vi "Teleop.vi"(10 "Match Info":T1={"Autonomous Elapsed Seconds"=0.0, "TeleOp Elapsed Seconds"=0.0, "Disabled Elapsed Seconds"=0.0, "Visited Autonomous"=FALSE, "Visited TeleOp"=FALSE, "Visited Disabled"=FALSE, "Autonomous Settings"={"Autonomous Style"=enum."Independent", "VI Refnum"=refnum}}, 11 "Call Context":T2) -> ()   [LabVIEW 2019]
doc: "This VI is called for each TeleOp packet received from the DS where the robot is not disabled. It is often used to read from the joysticks and update I/O or to update setpoints for timed control loops. It should complete and return within 20 milliseconds or it may miss DS packets."
uses:
  <vilib>/Rock Robotics/WPI/DriverStation/WPI_DriverStationDerivedRobotMode.ctl
  <vilib>/Rock Robotics/WPI/DriverStation/WPI_DriverStationMatch Info.ctl
  <vilib>/Rock Robotics/WPI/Utilities/WPI_GetSetVariantRefNum.vi
  <vilib>/Rock Robotics/Network Tables/NT Write Boolean Array.vi
  <vilib>/Rock Robotics/Network Tables/NT Write Numeric Array.vi
  <vilib>/Rock Robotics/Network Tables/NT Read Boolean.vi
  <vilib>/Rock Robotics/Network Tables/NT Read Number.vi
  <vilib>/Rock Robotics/Network Tables/NT Write Boolean.vi
  <vilib>/Rock Robotics/Network Tables/NT Write Number.vi
  <vilib>/Rock Robotics/Network Tables/NT Write String.vi
panel:
  out "Sample Slider 0":dbl(slide) scale=0.0..5.0
  out "Sample Boolean 1":bool
  out "Sample Boolean 0":bool
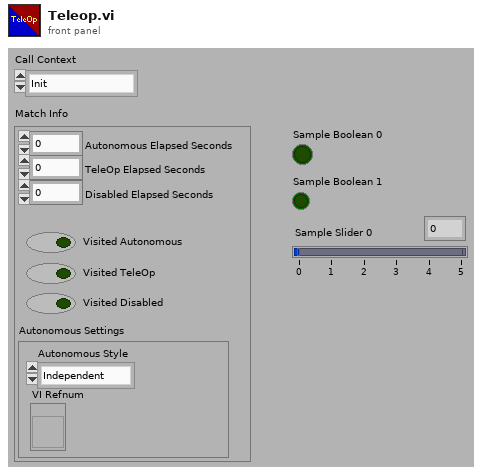
[diagram p1: front panel]
types:
  T1 = typedef "WPI_DriverStationMatch Info.ctl" = cluster{"Autonomous Elapsed Seconds":dbl, "TeleOp Elapsed Seconds":dbl, "Disabled Elapsed Seconds":dbl, "Visited Autonomous":bool, "Visited TeleOp":bool, "Visited Disabled":bool, "Autonomous Settings":cluster{"Autonomous Style":enum16{"Iterative", "Independent"}, "VI Refnum":refnum<vi>}}
  T2 = typedef "WPI_DriverStationDerivedRobotMode.ctl" = enum16{"Init", "Execute", "Stop"}
  T3 = typedef "WPI_JoystickDevRef.ctl" = cluster{"Device":T4}
  T4 = typedef "WPI_JoystickDeviceEnum.ctl" = enum16{"USB 0", "USB 1", "USB 2", "USB 3", "USB 4", "USB 5"}
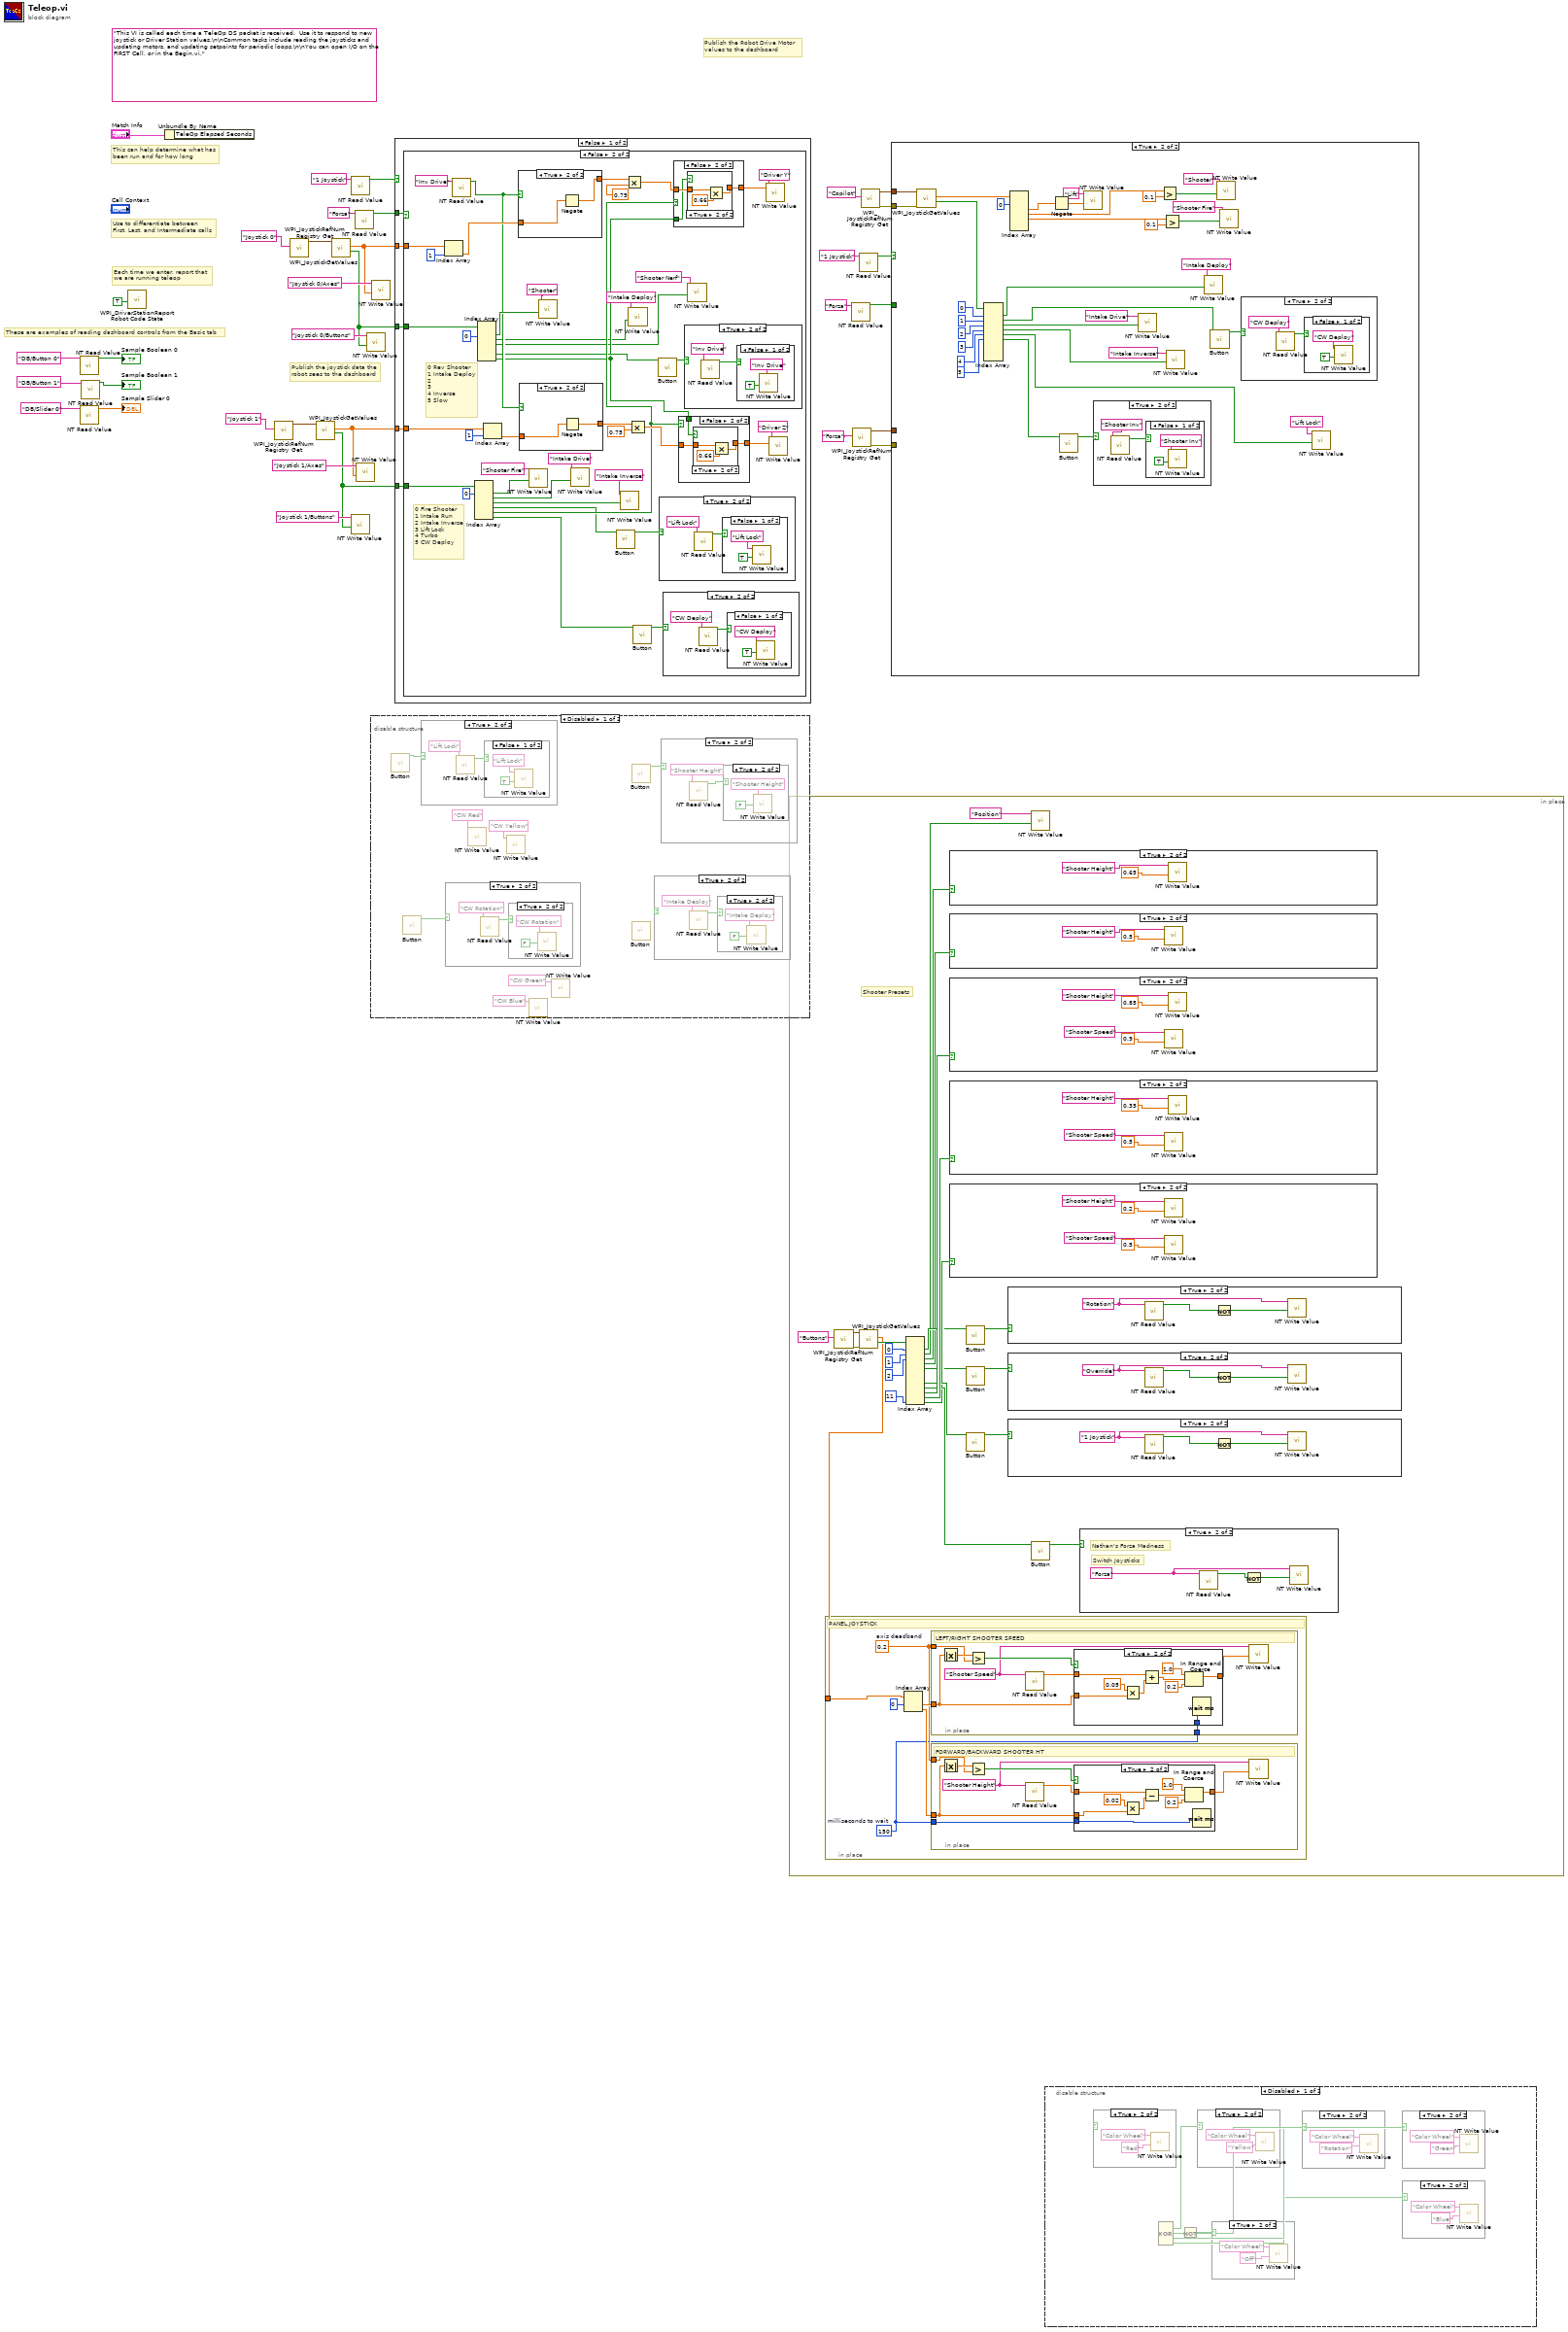
[diagram p0: block diagram]
diagram:
  (unwired) "This VI is called each time a TeleOp DS packet is received.  Use it to respond to new joystick or Driver Station values.\n\nCommon tasks include reading the joysticks and updating motors, and updating setpoints for periodic loops.\n\nYou can open I/O on the FIRST Call, or in the Begin.vi."
  # "These are examples of reading dashboard controls from the Basic tab"
  # "Publish the Robot Drive Motor\nvalues to the dashboard"
  # "Publish the joystick data the\nrobot sees to the dashboard"
  # "Each time we enter, report that\nwe are running teleop"
  # "Use to differentiate between\nFirst, Last, and Intermediate calls"
  # "This can help determine what has\nbeen run and for how long"
  n1 = call-poly <vilib>:"NT Read Value.vi"("Name"="DB/Button 0" ("refnum name")) -> ("Boolean"=→"Sample Boolean 0":bool)  [unwired: 9 in, 1 out]
  n2 = call-poly <vilib>:"NT Read Value.vi"("Name"="DB/Slider 0" ("refnum name")) -> ("Numeric"=→"Sample Slider 0":dbl)  [unwired: 9 in, 1 out]
  n3 = call-poly <vilib>:"NT Read Value.vi"("Name"="DB/Button 1" ("refnum name")) -> ("Boolean"=→"Sample Boolean 1":bool)  [unwired: 9 in, 1 out]
  n4 = call <vilib>:"WPI_DriverStationReport Robot Code State.vi"("TeleOp"=TRUE ("Autonomous")) -> ()  [unwired: 10 in, 1 out]
  n5 = Unbundle By Name("Match Info") -> ()  [unwired: 1 out]
  n6 = call <vilib>:"WPI_JoystickRefNum Registry Get.vi"("refnum name"="Joystick 1") -> ("JoystickDevRef"=w14:T3)  [unwired: 1 in, 9 out]
  n7 = call <vilib>:"WPI_JoystickRefNum Registry Get.vi"("refnum name"="Joystick 0") -> ("JoystickDevRef"=w32:T3)  [unwired: 1 in, 9 out]
  n8 = call <vilib>:"WPI_JoystickGetValues.vi"("JoystickDevRef"=w14) -> ("Buttons"=w10:bool[], "Axes"=w11:dbl[])  [unwired: 6 in, 3 out]
  n9 = call <vilib>:"WPI_JoystickGetValues.vi"("JoystickDevRef"=w32) -> ("Buttons"=w21:bool[], "Axes"=w28:dbl[])  [unwired: 6 in, 3 out]
  n10 = call-poly <vilib>:"NT Write Value.vi"("Boolean Array"=w10, "Name"="Joystick 1/Buttons") -> ()  [unwired: 9 in, 1 out]
  n11 = call-poly <vilib>:"NT Read Value.vi"("Name"="1 Joystick") -> ("Boolean"=w16:bool)  [unwired: 9 in, 1 out]
  n12 = call-poly <vilib>:"NT Read Value.vi"("Name"="Forza") -> ("Boolean"=w4:bool)  [unwired: 9 in, 1 out]
  n13 = call-poly <vilib>:"NT Write Value.vi"("Numeric Array"=w11, "Name"="Joystick 1/Axes") -> ()  [unwired: 9 in, 1 out]
  n14 = call-poly <vilib>:"NT Write Value.vi"("Boolean Array"=w21, "Name"="Joystick 0/Buttons") -> ()  [unwired: 9 in, 1 out]
  n15 = disable-structure shown="Disabled" {
    frame Disabled {
      n16 = call "Button.vi"() -> ("Button Pressed?"=w40:bool)  [unwired: 11 in]
      n17 = call "Button.vi"() -> ("Button Pressed?"=w35:bool)  [unwired: 11 in]
      n18 = case shown="True" w40 {
        frame False {
        }
        frame True {
          n19 = call-poly <vilib>:"NT Read Value.vi"("Name"="Lift Lock") -> ("Boolean"=w49:bool)  [unwired: 9 in, 1 out]
          n20 = case shown="False" w49 {
            frame False {
              n21 = call-poly <vilib>:"NT Write Value.vi"("Boolean"=TRUE, "Name"="Lift Lock") -> ()  [unwired: 9 in, 1 out]
            }
            frame True {
              n22 = call-poly <vilib>:"NT Write Value.vi"("Boolean"=FALSE, "Name"="Lift Lock") -> ()  [unwired: 9 in, 1 out]
            }
          }
        }
      }
      n23 = case shown="True" w35 {
        frame False {
        }
        frame True {
          n24 = call-poly <vilib>:"NT Read Value.vi"("Name"="CW Rotation") -> ("Boolean"=w43:bool)  [unwired: 9 in, 1 out]
          n25 = case shown="True" w43 {
            frame False {
              n26 = call-poly <vilib>:"NT Write Value.vi"("Boolean"=TRUE, "Name"="CW Rotation") -> ()  [unwired: 9 in, 1 out]
            }
            frame True {
              n27 = call-poly <vilib>:"NT Write Value.vi"("Boolean"=FALSE, "Name"="CW Rotation") -> ()  [unwired: 9 in, 1 out]
            }
          }
        }
      }
      n28 = call-poly <vilib>:"NT Write Value.vi"("Name"="CW Red") -> ()  [unwired: 10 in, 1 out]
      n29 = call-poly <vilib>:"NT Write Value.vi"("Name"="CW Yellow") -> ()  [unwired: 10 in, 1 out]
      n30 = call-poly <vilib>:"NT Write Value.vi"("Name"="CW Blue") -> ()  [unwired: 10 in, 1 out]
      n31 = call-poly <vilib>:"NT Write Value.vi"("Name"="CW Green") -> ()  [unwired: 10 in, 1 out]
      n32 = call "Button.vi"() -> ("Button Pressed?"=w42:bool)  [unwired: 11 in]
      n33 = call "Button.vi"() -> ()  [unwired: 11 in, 1 out]
      n34 = case shown="True" w41 {
        frame False {
        }
        frame True {
          n35 = call-poly <vilib>:"NT Read Value.vi"("Name"="Intake Deploy") -> ("Boolean"=w55:bool)  [unwired: 9 in, 1 out]
          n36 = case shown="True" w55 {
            frame False {
              n37 = call-poly <vilib>:"NT Write Value.vi"("Boolean"=TRUE, "Name"="Intake Deploy") -> ()  [unwired: 9 in, 1 out]
            }
            frame True {
              n38 = call-poly <vilib>:"NT Write Value.vi"("Boolean"=FALSE, "Name"="Intake Deploy") -> ()  [unwired: 9 in, 1 out]
            }
          }
        }
      }
      n39 = case shown="True" w42 {
        frame False {
        }
        frame True {
          n40 = call-poly <vilib>:"NT Read Value.vi"("Name"="Shooter Height") -> ("Boolean"=w61:bool)  [unwired: 9 in, 1 out]
          n41 = case shown="True" w61 {
            frame False {
              n42 = call-poly <vilib>:"NT Write Value.vi"("Boolean"=TRUE, "Name"="Shooter Height") -> ()  [unwired: 9 in, 1 out]
            }
            frame True {
              n43 = call-poly <vilib>:"NT Write Value.vi"("Boolean"=FALSE, "Name"="Shooter Height") -> ()  [unwired: 9 in, 1 out]
            }
          }
        }
      }
    }
    frame Enabled {
    }
  }
  n44 = call-poly <vilib>:"NT Write Value.vi"("Numeric Array"=w28, "Name"="Joystick 0/Axes") -> ()  [unwired: 9 in, 1 out]
  n45 = case shown="False" w16 {
    tunnel: w28 -> [w71 w179]
    tunnel: w21 -> [w70 w178]
    tunnel: w11 -> [w69 _]
    tunnel: w10 -> [w68 _]
    tunnel: w4 -> [w67 _]
    frame False {
      n46 = case shown="False" w67 {
        tunnel: w71 -> [_ w105]
        tunnel: w70 -> [_ w104]
        tunnel: w69 -> [_ w103]
        tunnel: w68 -> [_ w101]
        frame True {
        }
        frame False {
          # "0 Fire Shooter\n1 Intake Run\n2 Intake Inverse\n3 Lift Lock\n4 Turbo\n5 CW Deploy"
          # "0 Rev Shooter\n1 Intake Deploy\n2\n3\n4 Inverse\n5 Slow"
          n47 = Index Array(array=w105, index=1) -> (element=w110:dbl)
          n48 = call-poly <vilib>:"NT Read Value.vi"("Name"="Inv Drive") -> ("Boolean"=w84:bool)  [unwired: 9 in, 1 out]
          n49 = Index Array(array=w101, index #1=0 ("index")) -> (element #1=w92:bool, element #2=w89:bool, element #3=w77:bool, element #4=w78:bool, element #5=w83:bool, element #6=w86:bool)  [unwired: 5 in]
          n50 = Index Array(array=w104, index #1=0) -> (element #1=w88:bool, element #2=w74:bool, element #3=w72:bool, element #5=w81:bool, element #6=w80:bool)  [unwired: 5 in, 1 out]
          n51 = Index Array(array=w103, index=1) -> (element=w100:dbl)
          n52 = case shown="True" w84 {
            tunnel: w110 -> [w145 w147]
            tunnel: [w145 w146] -> w109
            frame False {
            }
            frame True {
              n53 = Negate(x=w147) -> (-x=w146:dbl)
            }
          }
          n54 = case shown="True" w84 {
            tunnel: w100 -> [w142 w144]
            tunnel: [w142 w143] -> w95
            frame False {
            }
            frame True {
              n55 = Negate(x=w144) -> (-x=w143:dbl)
            }
          }
          n56 = call-poly <vilib>:"NT Write Value.vi"("Boolean"=w92, "Name"="Shooter Fire") -> ()  [unwired: 9 in, 1 out]
          n57 = call-poly <vilib>:"NT Write Value.vi"("Boolean"=w88, "Name"="Shooter") -> ()  [unwired: 9 in, 1 out]
          n58 = call-poly <vilib>:"NT Write Value.vi"("Boolean"=w89, "Name"="Intake Drive") -> ()  [unwired: 9 in, 1 out]
          n59 = call "Button.vi"("Button In"=w78) -> ("Button Pressed?"=w79:bool)  [unwired: 10 in]
          n60 = call-poly <vilib>:"NT Write Value.vi"("Boolean"=w77, "Name"="Intake Inverse") -> ()  [unwired: 9 in, 1 out]
          n61 = Multiply(x=w109, y=0.75) -> (x*y=w108:dbl)
          n62 = call-poly <vilib>:"NT Write Value.vi"("Boolean"=w74, "Name"="Intake Deploy") -> ()  [unwired: 9 in, 1 out]
          n63 = Multiply(x=w95, y=0.75) -> (x*y=w98:dbl)
          n64 = call "Button.vi"("Button In"=w86) -> ("Button Pressed?"=w87:bool)  [unwired: 10 in]
          n65 = call "Button.vi"("Button In"=w81) -> ("Button Pressed?"=w82:bool)  [unwired: 10 in]
          n66 = case shown="True" w79 {
            frame False {
            }
            frame True {
              n67 = call-poly <vilib>:"NT Read Value.vi"("Name"="Lift Lock") -> ("Boolean"=w114:bool)  [unwired: 9 in, 1 out]
              n68 = case shown="False" w114 {
                frame False {
                  n69 = call-poly <vilib>:"NT Write Value.vi"("Boolean"=TRUE, "Name"="Lift Lock") -> ()  [unwired: 9 in, 1 out]
                }
                frame True {
                  n70 = call-poly <vilib>:"NT Write Value.vi"("Boolean"=FALSE, "Name"="Lift Lock") -> ()  [unwired: 9 in, 1 out]
                }
              }
            }
          }
          n71 = case shown="True" w87 {
            frame False {
            }
            frame True {
              n72 = call-poly <vilib>:"NT Read Value.vi"("Name"="CW Deploy") -> ("Boolean"=w126:bool)  [unwired: 9 in, 1 out]
              n73 = case shown="False" w126 {
                frame False {
                  n74 = call-poly <vilib>:"NT Write Value.vi"("Boolean"=TRUE, "Name"="CW Deploy") -> ()  [unwired: 9 in, 1 out]
                }
                frame True {
                  n75 = call-poly <vilib>:"NT Write Value.vi"("Boolean"=FALSE, "Name"="CW Deploy") -> ()  [unwired: 9 in, 1 out]
                }
              }
            }
          }
          n76 = case shown="False" w83 {
            tunnel: w108 -> [w149 w153]
            tunnel: [w148 w152] -> w107
            tunnel: w80 -> [_ w151]
            frame True {
              n77 = Multiply(x=w149, y=1.33) -> (x*y=w148:dbl)
            }
            frame False {
              n78 = case shown="True" w151 {
                tunnel: w153 -> [w154 w156]
                tunnel: [w154 w155] -> w152
                frame False {
                }
                frame True {
                  n79 = Multiply(x=w156, y=0.66) -> (x*y=w155:dbl)
                }
              }
            }
          }
          n80 = case shown="False" w83 {
            tunnel: w98 -> [w133 w137]
            tunnel: [w132 w136] -> w97
            tunnel: w80 -> [_ w135]
            frame True {
              n81 = Multiply(x=w133, y=1.33) -> (x*y=w132:dbl)
            }
            frame False {
              n82 = case shown="True" w135 {
                tunnel: w137 -> [w138 w140]
                tunnel: [w138 w139] -> w136
                frame False {
                }
                frame True {
                  n83 = Multiply(x=w140, y=0.66) -> (x*y=w139:dbl)
                }
              }
            }
          }
          n84 = case shown="True" w82 {
            frame False {
            }
            frame True {
              n85 = call-poly <vilib>:"NT Read Value.vi"("Name"="Inv Drive") -> ("Boolean"=w120:bool)  [unwired: 9 in, 1 out]
              n86 = case shown="False" w120 {
                frame False {
                  n87 = call-poly <vilib>:"NT Write Value.vi"("Boolean"=TRUE, "Name"="Inv Drive") -> ()  [unwired: 9 in, 1 out]
                }
                frame True {
                  n88 = call-poly <vilib>:"NT Write Value.vi"("Boolean"=FALSE, "Name"="Inv Drive") -> ()  [unwired: 9 in, 1 out]
                }
              }
            }
          }
          n89 = call-poly <vilib>:"NT Write Value.vi"("Boolean"=w72, "Name"="Shooter Nerf") -> ()  [unwired: 9 in, 1 out]
          n90 = call-poly <vilib>:"NT Write Value.vi"("Numeric"=w107, "Name"="Driver Y") -> ()  [unwired: 9 in, 1 out]
          n91 = call-poly <vilib>:"NT Write Value.vi"("Numeric"=w97, "Name"="Driver Z") -> ()  [unwired: 9 in, 1 out]
        }
      }
    }
    frame True {
      # "0 Turbo\n1 Slow\n2\n3\n4 Inverse\n5"
      n92 = Index Array(array=w179, index #1=1, index #2=3) -> (element #1=w173:dbl, element #2=w168:dbl)
      n93 = Index Array(array=w178, index #1=0) -> (element #1=w162:bool, element #2=w163:bool, element #5=w160:bool)  [unwired: 5 in, 3 out]
      n94 = call-poly <vilib>:"NT Read Value.vi"("Name"="Inv Drive") -> ("Boolean"=w159:bool)  [unwired: 9 in, 1 out]
      n95 = Multiply(x=w168, y=0.5) -> (x*y=w169:dbl)
      n96 = case shown="True" w159 {
        tunnel: w173 -> [w196 w198]
        tunnel: [w196 w197] -> w172
        frame False {
        }
        frame True {
          n97 = Negate(x=w198) -> (-x=w197:dbl)
        }
      }
      n98 = case shown="True" w162 {
        tunnel: [w186 w190] -> w167
        tunnel: w169 -> [w187 w191]
        tunnel: w163 -> [_ w189]
        frame True {
          n99 = Multiply(x=w187, y=1.33) -> (x*y=w186:dbl)
        }
        frame False {
          n100 = case shown="True" w189 {
            tunnel: [w192 w194] -> w190
            tunnel: w191 -> [w192 w193]
            frame False {
            }
            frame True {
              n101 = Multiply(x=w193, y=0.66) -> (x*y=w194:dbl)
            }
          }
        }
      }
      n102 = call "Button.vi"("Button In"=w160) -> ("Button Pressed?"=w161:bool)  [unwired: 10 in]
      n103 = case shown="True" w161 {
        frame False {
        }
        frame True {
          n104 = call-poly <vilib>:"NT Read Value.vi"("Name"="Inv Drive") -> ("Boolean"=w180:bool)  [unwired: 9 in, 1 out]
          n105 = case shown="False" w180 {
            frame False {
              n106 = call-poly <vilib>:"NT Write Value.vi"("Boolean"=TRUE, "Name"="Inv Drive") -> ()  [unwired: 9 in, 1 out]
            }
            frame True {
              n107 = call-poly <vilib>:"NT Write Value.vi"("Boolean"=FALSE, "Name"="Inv Drive") -> ()  [unwired: 9 in, 1 out]
            }
          }
        }
      }
      n108 = Multiply(x=w172, y=0.6) -> (x*y=w171:dbl)
      n109 = call-poly <vilib>:"NT Write Value.vi"("Numeric"=w167, "Name"="Driver Z") -> ()  [unwired: 9 in, 1 out]
      n110 = case shown="True" w162 {
        tunnel: w171 -> [w200 w204]
        tunnel: [w199 w203] -> w165
        tunnel: w163 -> [_ w202]
        frame True {
          n111 = Multiply(x=w200, y=1.33) -> (x*y=w199:dbl)
        }
        frame False {
          n112 = case shown="False" w202 {
            tunnel: w204 -> [w205 w207]
            tunnel: [w205 w206] -> w203
            frame False {
            }
            frame True {
              n113 = Multiply(x=w207, y=0.66) -> (x*y=w206:dbl)
            }
          }
        }
      }
      n114 = call-poly <vilib>:"NT Write Value.vi"("Numeric"=w165, "Name"="Driver Y") -> ()  [unwired: 9 in, 1 out]
    }
  }
  n115 = in-place {
    # "Shooter Presets"
    n116 = call <vilib>:"WPI_JoystickRefNum Registry Get.vi"("refnum name"="Buttons") -> ("error out"=w232:errorcluster, "JoystickDevRef"=w231:T3)  [unwired: 9 in]
    n117 = call <vilib>:"WPI_JoystickGetValues.vi"("error in (no error)"=w232, "JoystickDevRef"=w231) -> ("Buttons"=w229:bool[], "Axes"=w209:dbl[])  [unwired: 5 in, 3 out]
    n118 = in-place {
      in-place-border: w209 -> [w238]
      w233 = u32 150  # milliseconds to wait
      w234 = 0.2  # axis deadband
      # "PANEL JOYSTICK"
      n119 = Index Array(array=w238, index #1=0 ("index")) -> (element #1=w236:dbl, element #2=w235:dbl)  [unwired: 1 in]
      n120 = in-place {
        in-place-border: w236 -> [w262]
        in-place-border: w234 -> [w258]
        in-place-border: w233 -> [w257]
        w260 = "Shooter Speed"
        # "LEFT/RIGHT SHOOTER SPEED"
        n121 = Absolute Value(x=w262) -> (abs(x)=w263:dbl)
        n122 = Greater?(x=w263, y=w258) -> (0:w264:bool)
        n123 = call-poly <vilib>:"NT Read Value.vi"("Name"=w260) -> ("Numeric"=w259:dbl)  [unwired: 9 in, 1 out]
        n124 = case shown="True" w264 {
          tunnel: w262 -> [_ w271]
          tunnel: [w265 w268] -> w261
          tunnel: w259 -> [w265 w267]
          tunnel: w257 -> [_ w266]
          frame False {
          }
          frame True {
            n125 = Multiply(x=0.05 ("y"), y=w271) -> (x*y=w272:dbl)
            n126 = Add(x=w267, y=w272) -> (x+y=w274:dbl)
            n127 = In Range and Coerce(upper limit=1.0, x=w274, lower limit=0.2) -> (coerced(x)=w268:dbl)  [unwired: 1 out]
            n128 = Wait (ms)(milliseconds to wait=w266) -> ()  [unwired: 1 out]
          }
        }
        n129 = call-poly <vilib>:"NT Write Value.vi"("Numeric"=w261, "Name"=w260) -> ()  [unwired: 9 in, 1 out]
      }
      n130 = in-place {
        in-place-border: w235 -> [w244]
        in-place-border: w234 -> [w240]
        in-place-border: w233 -> [w239]
        w243 = "Shooter Height"
        # "FORWARD/BACKWARD SHOOTER HT"
        n131 = Absolute Value(x=w244) -> (abs(x)=w245:dbl)
        n132 = Greater?(x=w245, y=w240) -> (0:w246:bool)
        n133 = call-poly <vilib>:"NT Read Value.vi"("Name"=w243) -> ("Numeric"=w242:dbl)  [unwired: 9 in, 1 out]
        n134 = case shown="True" w246 {
          tunnel: w244 -> [_ w253]
          tunnel: w242 -> [w247 w250]
          tunnel: [w247 w249] -> w241
          tunnel: w239 -> [_ w248]
          frame False {
          }
          frame True {
            n135 = Multiply(x=0.02 ("y"), y=w253) -> (x*y=w254:dbl)
            n136 = Subtract(x=w250, y=w254) -> (x-y=w256:dbl)
            n137 = In Range and Coerce(upper limit=1.0, x=w256, lower limit=0.2) -> (coerced(x)=w249:dbl)  [unwired: 1 out]
            n138 = Wait (ms)(milliseconds to wait=w248) -> ()  [unwired: 1 out]
          }
        }
        n139 = call-poly <vilib>:"NT Write Value.vi"("Numeric"=w241, "Name"=w243) -> ()  [unwired: 9 in, 1 out]
      }
    }
    n140 = Index Array(array=w229, index #1=0 ("index"), index #2=1 ("index"), index #3=2 ("index"), index #12=11 ("index")) -> (element #1=w215:bool, element #2=w213:bool, element #3=w211:bool, element #4=w210:bool, element #5=w212:bool, element #8=w224:bool, element #9=w222:bool, element #10=w226:bool, element #11=w227:bool, element #12=w218:bool)  [unwired: 8 in, 2 out]
    n141 = case shown="True" w211 {
      frame False {
      }
      frame True {
        n142 = call-poly <vilib>:"NT Write Value.vi"("Numeric"=0.65, "Name"="Shooter Height") -> ()  [unwired: 9 in, 1 out]
      }
    }
    n143 = case shown="True" w210 {
      frame False {
      }
      frame True {
        n144 = call-poly <vilib>:"NT Write Value.vi"("Numeric"=0.5, "Name"="Shooter Height") -> ()  [unwired: 9 in, 1 out]
      }
    }
    n145 = case shown="True" w226 {
      frame False {
      }
      frame True {
        n146 = call-poly <vilib>:"NT Write Value.vi"("Numeric"=0.9, "Name"="Shooter Speed") -> ()  [unwired: 9 in, 1 out]
        n147 = call-poly <vilib>:"NT Write Value.vi"("Numeric"=0.85, "Name"="Shooter Height") -> ()  [unwired: 9 in, 1 out]
      }
    }
    n148 = case shown="True" w227 {
      frame False {
      }
      frame True {
        n149 = call-poly <vilib>:"NT Write Value.vi"("Numeric"=0.5, "Name"="Shooter Speed") -> ()  [unwired: 9 in, 1 out]
        n150 = call-poly <vilib>:"NT Write Value.vi"("Numeric"=0.35, "Name"="Shooter Height") -> ()  [unwired: 9 in, 1 out]
      }
    }
    n151 = case shown="True" w218 {
      frame False {
      }
      frame True {
        n152 = call-poly <vilib>:"NT Write Value.vi"("Numeric"=0.2, "Name"="Shooter Height") -> ()  [unwired: 9 in, 1 out]
        n153 = call-poly <vilib>:"NT Write Value.vi"("Numeric"=0.5, "Name"="Shooter Speed") -> ()  [unwired: 9 in, 1 out]
      }
    }
    n154 = call "Button.vi"("Button In"=w215) -> ("Button Pressed?"=w217:bool)  [unwired: 10 in]
    n155 = call "Button.vi"("Button In"=w212) -> ("Button Pressed?"=w216:bool)  [unwired: 10 in]
    n156 = call "Button.vi"("Button In"=w224) -> ("Button Pressed?"=w225:bool)  [unwired: 10 in]
    n157 = case shown="True" w217 {
      frame False {
      }
      frame True {
        w284 = "Rotation"
        n158 = call-poly <vilib>:"NT Read Value.vi"("Name"=w284) -> ("Boolean"=w283:bool)  [unwired: 9 in, 1 out]
        n159 = Not(x=w283) -> (.not. x?=w282:bool)
        n160 = call-poly <vilib>:"NT Write Value.vi"("Boolean"=w282, "Name"=w284) -> ()  [unwired: 9 in, 1 out]
      }
    }
    n161 = case shown="True" w216 {
      frame False {
      }
      frame True {
        w280 = "Override"
        n162 = call-poly <vilib>:"NT Read Value.vi"("Name"=w280) -> ("Boolean"=w281:bool)  [unwired: 9 in, 1 out]
        n163 = Not(x=w281) -> (.not. x?=w279:bool)
        n164 = call-poly <vilib>:"NT Write Value.vi"("Boolean"=w279, "Name"=w280) -> ()  [unwired: 9 in, 1 out]
      }
    }
    n165 = case shown="True" w225 {
      frame False {
      }
      frame True {
        w294 = "1 Joystick"
        n166 = call-poly <vilib>:"NT Read Value.vi"("Name"=w294) -> ("Boolean"=w293:bool)  [unwired: 9 in, 1 out]
        n167 = Not(x=w293) -> (.not. x?=w292:bool)
        n168 = call-poly <vilib>:"NT Write Value.vi"("Boolean"=w292, "Name"=w294) -> ()  [unwired: 9 in, 1 out]
      }
    }
    n169 = call-poly <vilib>:"NT Write Value.vi"("Boolean"=w213, "Name"="Position") -> ()  [unwired: 9 in, 1 out]
    n170 = call "Button.vi"("Button In"=w222) -> ("Button Pressed?"=w223:bool)  [unwired: 10 in]
    n171 = case shown="True" w223 {
      frame False {
      }
      frame True {
        w290 = "Forza"
        # "Switch Joysticks"
        # "Nathan's Forza Madness"
        n172 = call-poly <vilib>:"NT Read Value.vi"("Name"=w290) -> ("Boolean"=w291:bool)  [unwired: 9 in, 1 out]
        n173 = Not(x=w291) -> (.not. x?=w289:bool)
        n174 = call-poly <vilib>:"NT Write Value.vi"("Boolean"=w289, "Name"=w290) -> ()  [unwired: 9 in, 1 out]
      }
    }
  }
  n175 = call-poly <vilib>:"NT Read Value.vi"("Name"="Forza") -> ("Boolean"=w6:bool)  [unwired: 9 in, 1 out]
  n176 = call <vilib>:"WPI_JoystickRefNum Registry Get.vi"("refnum name"="Forza") -> ("error out"=w1:errorcluster, "JoystickDevRef"=w2:T3)  [unwired: 9 in]
  n177 = call-poly <vilib>:"NT Read Value.vi"("Name"="1 Joystick") -> ("Boolean"=w8:bool)  [unwired: 9 in, 1 out]
  n178 = call <vilib>:"WPI_JoystickRefNum Registry Get.vi"("refnum name"="Copilot") -> ("error out"=w20:errorcluster, "JoystickDevRef"=w19:T3)  [unwired: 9 in]
  n179 = case shown="True" w8 {
    tunnel: w20 -> [w306 w456]
    tunnel: w19 -> [w307 w455]
    tunnel: w6 -> [w305 _]
    tunnel: w2 -> [w304 _]
    tunnel: w1 -> [w303 _]
    frame False {
      n180 = case shown="True" w305 {
        tunnel: w307 -> [_ w367]
        tunnel: w306 -> [_ w366]
        tunnel: w304 -> [_ w360]
        tunnel: w303 -> [_ w359]
        frame False {
        }
        frame True {
          n181 = call <vilib>:"WPI_JoystickGetValues.vi"("error in (no error)"=w359, "JoystickDevRef"=w360) -> ("Buttons"=w364:bool[], "Axes"=w365:dbl[])  [unwired: 5 in, 3 out]
          n182 = call <vilib>:"WPI_JoystickGetValues.vi"("error in (no error)"=w366, "JoystickDevRef"=w367) -> ("Buttons"=w336:bool[], "Axes"=w337:dbl[])  [unwired: 5 in, 3 out]
          n183 = Index Array(array=w336, index #1=0, index #2=1, index #3=2, index #4=3) -> (element #1=w319:bool, element #2=w346:bool, element #3=w347:bool, element #4=w322:bool, element #5=w321:bool, element #6=w310:bool)  [unwired: 6 in, 4 out]
          n184 = Index Array(array=w337, index #1=0 ("index")) -> (element #2=w342:dbl, element #3=w352:dbl, element #4=w338:dbl)  [unwired: 5 in, 3 out]
          n185 = Index Array(array=w364, index #1=0 ("index")) -> (element #1=w316:bool, element #2=w317:bool, element #5=w314:bool)  [unwired: 9 in, 7 out]
          n186 = Index Array(array=w365, index #1=0 ("index")) -> (element #1=w326:dbl, element #3=w362:dbl, element #4=w335:dbl)  [unwired: 5 in, 3 out]
          n187 = Negate(x=w342) -> (-x=w343:dbl)
          n188 = call-poly <vilib>:"NT Write Value.vi"("Numeric"=w343, "Name"="Lift") -> ()  [unwired: 9 in, 1 out]
          n189 = Negate(x=w362) -> (-x=w361:dbl)
          n190 = Add(x=w361, y=w335) -> (x+y=w327:dbl)
          n191 = call-poly <vilib>:"NT Read Value.vi"("Name"="Override") -> ("Boolean"=w308:bool)  [unwired: 9 in, 1 out]
          n192 = Multiply(x=0.7, y=w326) -> (x*y=w332:dbl)
          n193 = case shown="False" w308 {
            tunnel: w332 -> [w369 w374]
            tunnel: [w368 w373] -> w331
            tunnel: w317 -> [_ w372]
            tunnel: w316 -> [_ w371]
            frame True {
              n194 = Multiply(x=w369, y=0.3) -> (x*y=w368:dbl)
            }
            frame False {
              n195 = case shown="False" w371 {
                tunnel: [w375 w379] -> w373
                tunnel: w374 -> [w376 w380]
                tunnel: w372 -> [_ w378]
                frame True {
                  n196 = Multiply(x=w376, y=0.5) -> (x*y=w375:dbl)
                }
                frame False {
                  n197 = case shown="False" w378 {
                    tunnel: [w381 w383] -> w379
                    tunnel: w380 -> [w381 w382]
                    frame False {
                    }
                    frame True {
                      n198 = Multiply(x=w382, y=1.33) -> (x*y=w383:dbl)
                    }
                  }
                }
              }
            }
          }
          n199 = call-poly <vilib>:"NT Read Value.vi"("Name"="Inv Drive") -> ("Boolean"=w312:bool)  [unwired: 9 in, 1 out]
          n200 = call-poly <vilib>:"NT Write Value.vi"("Boolean"=w347, "Name"="Intake Drive") -> ()  [unwired: 9 in, 1 out]
          n201 = Greater?(x=w352, y=0.1) -> (0:w349:bool)
          n202 = Greater?(x=w338, y=0.1) -> (0:w339:bool)
          n203 = case shown="True" w312 {
            tunnel: [w414 w416] -> w334
            tunnel: w327 -> [w414 w415]
            frame False {
            }
            frame True {
              n204 = Negate(x=w415) -> (-x=w416:dbl)
            }
          }
          n205 = call-poly <vilib>:"NT Write Value.vi"("Boolean"=w321, "Name"="Lift Lock") -> ()  [unwired: 9 in, 1 out]
          n206 = call-poly <vilib>:"NT Write Value.vi"("Boolean"=w349, "Name"="Shooter") -> ()  [unwired: 9 in, 1 out]
          n207 = call-poly <vilib>:"NT Write Value.vi"("Boolean"=w339, "Name"="Shooter Fire") -> ()  [unwired: 9 in, 1 out]
          n208 = call-poly <vilib>:"NT Write Value.vi"("Boolean"=w319, "Name"="Intake Deploy") -> ()  [unwired: 9 in, 1 out]
          n209 = call "Button.vi"("Button In"=w346) -> ("Button Pressed?"=w345:bool)  [unwired: 10 in]
          n210 = call-poly <vilib>:"NT Write Value.vi"("Boolean"=w322, "Name"="Intake Inverse") -> ()  [unwired: 9 in, 1 out]
          n211 = call-poly <vilib>:"NT Write Value.vi"("Numeric"=w331, "Name"="Driver Z") -> ()  [unwired: 9 in, 1 out]
          n212 = call "Button.vi"("Button In"=w310) -> ("Button Pressed?"=w311:bool)  [unwired: 10 in]
          n213 = Multiply(x=w334, y=0.6) -> (x*y=w333:dbl)
          n214 = call "Button.vi"("Button In"=w314) -> ("Button Pressed?"=w315:bool)  [unwired: 10 in]
          n215 = case shown="True" w345 {
            frame False {
            }
            frame True {
              n216 = call-poly <vilib>:"NT Read Value.vi"("Name"="CW Deploy") -> ("Boolean"=w417:bool)  [unwired: 9 in, 1 out]
              n217 = case shown="False" w417 {
                frame False {
                  n218 = call-poly <vilib>:"NT Write Value.vi"("Boolean"=TRUE, "Name"="CW Deploy") -> ()  [unwired: 9 in, 1 out]
                }
                frame True {
                  n219 = call-poly <vilib>:"NT Write Value.vi"("Boolean"=FALSE, "Name"="CW Deploy") -> ()  [unwired: 9 in, 1 out]
                }
              }
            }
          }
          n220 = case shown="True" w311 {
            frame False {
            }
            frame True {
              n221 = call-poly <vilib>:"NT Read Value.vi"("Name"="Shooter Inv") -> ("Boolean"=w402:bool)  [unwired: 9 in, 1 out]
              n222 = case shown="False" w402 {
                frame False {
                  n223 = call-poly <vilib>:"NT Write Value.vi"("Boolean"=TRUE, "Name"="Shooter Inv") -> ()  [unwired: 9 in, 1 out]
                }
                frame True {
                  n224 = call-poly <vilib>:"NT Write Value.vi"("Boolean"=FALSE, "Name"="Shooter Inv") -> ()  [unwired: 9 in, 1 out]
                }
              }
            }
          }
          n225 = case shown="False" w308 {
            tunnel: w333 -> [w385 w391]
            tunnel: [w386 w390] -> w329
            tunnel: w317 -> [_ w389]
            tunnel: w316 -> [_ w388]
            frame True {
              n226 = Multiply(x=w385, y=0.3) -> (x*y=w386:dbl)
            }
            frame False {
              n227 = case shown="False" w388 {
                tunnel: w391 -> [w393 w397]
                tunnel: [w392 w396] -> w390
                tunnel: w389 -> [_ w395]
                frame True {
                  n228 = Multiply(x=w393, y=0.5) -> (x*y=w392:dbl)
                }
                frame False {
                  n229 = case shown="False" w395 {
                    tunnel: w397 -> [w398 w400]
                    tunnel: [w398 w399] -> w396
                    frame False {
                    }
                    frame True {
                      n230 = Multiply(x=w400, y=1.33) -> (x*y=w399:dbl)
                    }
                  }
                }
              }
            }
          }
          n231 = case shown="True" w315 {
            frame False {
            }
            frame True {
              n232 = call-poly <vilib>:"NT Read Value.vi"("Name"="Inv Drive") -> ("Boolean"=w408:bool)  [unwired: 9 in, 1 out]
              n233 = case shown="False" w408 {
                frame False {
                  n234 = call-poly <vilib>:"NT Write Value.vi"("Boolean"=TRUE, "Name"="Inv Drive") -> ()  [unwired: 9 in, 1 out]
                }
                frame True {
                  n235 = call-poly <vilib>:"NT Write Value.vi"("Boolean"=FALSE, "Name"="Inv Drive") -> ()  [unwired: 9 in, 1 out]
                }
              }
            }
          }
          n236 = call-poly <vilib>:"NT Write Value.vi"("Numeric"=w329, "Name"="Driver Y") -> ()  [unwired: 9 in, 1 out]
        }
      }
    }
    frame True {
      n237 = call <vilib>:"WPI_JoystickGetValues.vi"("error in (no error)"=w456, "JoystickDevRef"=w455) -> ("Buttons"=w453:bool[], "Axes"=w454:dbl[])  [unwired: 5 in, 3 out]
      n238 = Index Array(array=w453, index #1=0, index #2=1, index #3=2, index #4=3, index #5=4 ("index"), index #6=5 ("index")) -> (element #1=w427:bool, element #2=w441:bool, element #3=w442:bool, element #4=w431:bool, element #5=w426:bool, element #6=w423:bool)  [unwired: 4 in, 4 out]
      n239 = Index Array(array=w454, index #1=0 ("index")) -> (element #2=w437:dbl, element #3=w447:dbl, element #4=w433:dbl)  [unwired: 5 in, 3 out]
      n240 = Negate(x=w437) -> (-x=w438:dbl)
      n241 = call "Button.vi"("Button In"=w423) -> ("Button Pressed?"=w424:bool)  [unwired: 10 in]
      n242 = call-poly <vilib>:"NT Write Value.vi"("Numeric"=w438, "Name"="Lift") -> ()  [unwired: 9 in, 1 out]
      n243 = case shown="True" w424 {
        frame False {
        }
        frame True {
          n244 = call-poly <vilib>:"NT Read Value.vi"("Name"="Shooter Inv") -> ("Boolean"=w457:bool)  [unwired: 9 in, 1 out]
          n245 = case shown="False" w457 {
            frame False {
              n246 = call-poly <vilib>:"NT Write Value.vi"("Boolean"=TRUE, "Name"="Shooter Inv") -> ()  [unwired: 9 in, 1 out]
            }
            frame True {
              n247 = call-poly <vilib>:"NT Write Value.vi"("Boolean"=FALSE, "Name"="Shooter Inv") -> ()  [unwired: 9 in, 1 out]
            }
          }
        }
      }
      n248 = call-poly <vilib>:"NT Write Value.vi"("Boolean"=w442, "Name"="Intake Drive") -> ()  [unwired: 9 in, 1 out]
      n249 = Greater?(x=w447, y=0.1) -> (0:w444:bool)
      n250 = Greater?(x=w433, y=0.1) -> (0:w434:bool)
      n251 = call-poly <vilib>:"NT Write Value.vi"("Boolean"=w431, "Name"="Intake Inverse") -> ()  [unwired: 9 in, 1 out]
      n252 = call-poly <vilib>:"NT Write Value.vi"("Boolean"=w427, "Name"="Intake Deploy") -> ()  [unwired: 9 in, 1 out]
      n253 = call "Button.vi"("Button In"=w441) -> ("Button Pressed?"=w440:bool)  [unwired: 10 in]
      n254 = call-poly <vilib>:"NT Write Value.vi"("Boolean"=w444, "Name"="Shooter") -> ()  [unwired: 9 in, 1 out]
      n255 = call-poly <vilib>:"NT Write Value.vi"("Boolean"=w434, "Name"="Shooter Fire") -> ()  [unwired: 9 in, 1 out]
      n256 = case shown="True" w440 {
        frame False {
        }
        frame True {
          n257 = call-poly <vilib>:"NT Read Value.vi"("Name"="CW Deploy") -> ("Boolean"=w463:bool)  [unwired: 9 in, 1 out]
          n258 = case shown="False" w463 {
            frame False {
              n259 = call-poly <vilib>:"NT Write Value.vi"("Boolean"=TRUE, "Name"="CW Deploy") -> ()  [unwired: 9 in, 1 out]
            }
            frame True {
              n260 = call-poly <vilib>:"NT Write Value.vi"("Boolean"=FALSE, "Name"="CW Deploy") -> ()  [unwired: 9 in, 1 out]
            }
          }
        }
      }
      n261 = call-poly <vilib>:"NT Write Value.vi"("Boolean"=w426, "Name"="Lift Lock") -> ()  [unwired: 9 in, 1 out]
    }
  }
  n262 = disable-structure shown="Disabled" {
    frame Disabled {
      n263 = case shown="True" w473 {
        frame False {
        }
        frame True {
          n264 = call-poly <vilib>:"NT Write Value.vi"("String"="Red", "Name"="Color Wheel") -> ()  [unwired: 9 in, 1 out]
        }
      }
      n265 = case shown="True" w476 {
        frame False {
        }
        frame True {
          n266 = call-poly <vilib>:"NT Write Value.vi"("String"="Yellow", "Name"="Color Wheel") -> ()  [unwired: 9 in, 1 out]
        }
      }
      n267 = case shown="True" w475 {
        frame False {
        }
        frame True {
          n268 = call-poly <vilib>:"NT Write Value.vi"("String"="Rotation", "Name"="Color Wheel") -> ()  [unwired: 9 in, 1 out]
        }
      }
      n269 = case shown="True" w470 {
        frame False {
        }
        frame True {
          n270 = call-poly <vilib>:"NT Write Value.vi"("String"="Green", "Name"="Color Wheel") -> ()  [unwired: 9 in, 1 out]
        }
      }
      n271 = case shown="True" w469 {
        frame False {
        }
        frame True {
          n272 = call-poly <vilib>:"NT Write Value.vi"("String"="Blue", "Name"="Color Wheel") -> ()  [unwired: 9 in, 1 out]
        }
      }
      n273 = Compound Arithmetic op=XOR(w476, w475, w470, w469) -> (w472:bool, w474:bool)
      n274 = Not(x=w472) -> (.not. x?=w471:bool)
      n275 = case shown="True" w471 {
        frame False {
        }
        frame True {
          n276 = call-poly <vilib>:"NT Write Value.vi"("String"="Off", "Name"="Color Wheel") -> ()  [unwired: 9 in, 1 out]
        }
      }
    }
    frame Enabled {
    }
  }
